vi "iPhone Receive Loop.vi"   [LabVIEW 2015]
uses:
  Global Data.vi
types:
  T1 = cluster{"Accel X":dbl, "Accel Y":dbl, "Accel Z":dbl, "Gyro X":dbl, "Gyro Y":dbl, "Gyro Z":dbl}
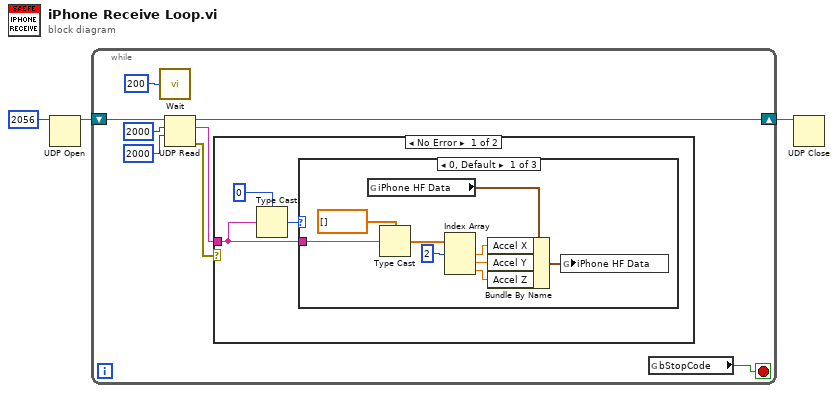
[diagram p0: block diagram]
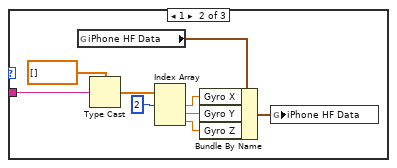
[diagram p2: hidden frame]
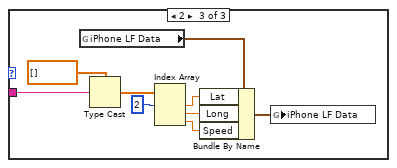
[diagram p3: hidden frame]
diagram:
  n1 = UDP Open(11:u16 2056 ("port")) -> (port=w1:refnum<k16>)  [unwired: 4 in, 2 out]
  n2 = while {
    shift-right: [w10] -> w3
    shift-left: w1 -> [w11]
    stop <- w5 stop-if-true
    n3 = call "Wait"("Count(uSec)"=u32 200) -> ()  [unwired: 1 out]
    n4 = UDP Read(connection ID=w11, max size (548)=2000, timeout ms (25000)=2000) -> (data out=w6:string, error out=w7:errorcluster, 3:w10:refnum<k16>)  [unwired: 1 in, 2 out]
    n5 = case shown="No Error" w7 {
      tunnel: w6 -> [w12 _]
      frame No Error {
        n6 = Type Cast(type=u8 0, x=w12) -> (*(type *) &x=w13:u8)
        n7 = case shown="0, Default" w13 {
          tunnel: w12 -> [w21 w30 w39]
          frame 0, Default {
            n8 = global read "Global Data.vi" "iPhone HF Data"() -> (w23:T1)
            n9 = Type Cast(type=dbl[] [], x=w21) -> (*(type *) &x=w19:dbl[])
            n10 = Index Array(array=w19, index #1=2 ("index")) -> (element #1=w17:dbl, element #2=w16:dbl, element #3=w15:dbl)  [unwired: 2 in]
            n11 = Bundle By Name(cluster=w23, "Accel X"=w17, "Accel Y"=w16, "Accel Z"=w15) -> (w22:T1)
            n12 = global write "Global Data.vi" "iPhone HF Data"(w22) -> ()
          }
          frame 1 {
            n13 = global read "Global Data.vi" "iPhone HF Data"() -> (w32:T1)
            n14 = Type Cast(type=dbl[] [], x=w30) -> (*(type *) &x=w28:dbl[])
            n15 = Index Array(array=w28, index #1=2 ("index")) -> (element #1=w26:dbl, element #2=w25:dbl, element #3=w24:dbl)  [unwired: 2 in]
            n16 = Bundle By Name(cluster=w32, "Gyro X"=w26, "Gyro Y"=w25, "Gyro Z"=w24) -> (w31:T1)
            n17 = global write "Global Data.vi" "iPhone HF Data"(w31) -> ()
          }
          frame 2 {
            n18 = global read "Global Data.vi" "iPhone LF Data"() -> (w41:cluster{"Lat":dbl, "Long":dbl, "Speed":dbl})
            n19 = Type Cast(type=dbl[] [], x=w39) -> (*(type *) &x=w37:dbl[])
            n20 = Index Array(array=w37, index #1=2 ("index")) -> (element #1=w35:dbl, element #2=w34:dbl, element #3=w33:dbl)  [unwired: 2 in]
            n21 = Bundle By Name(cluster=w41, "Lat"=w35, "Long"=w34, "Speed"=w33) -> (w40:cluster{"Lat":dbl, "Long":dbl, "Speed":dbl})
            n22 = global write "Global Data.vi" "iPhone LF Data"(w40) -> ()
          }
        }
      }
      frame Error {
      }
    }
    n23 = global read "Global Data.vi" "bStopCode"() -> (w5:bool)
  }
  n24 = UDP Close(connection ID=w3) -> ()  [unwired: 1 in, 2 out]
